vi "AMX-电源尾正面标签1检测参数读取.vi"(7 "error in (no error)":errorcluster caption="错误输入（无错误）", 10 "基路径":path) -> (0 "error out":errorcluster caption="错误输出", 1 "UI电源线尾正面标签1参数":T2={"Rectangle"={"Left"=0, "Top"=0, "Right"=0, "Bottom"=0, "Rotation"=0.0}, "Algorithm "=2, "Parameters"={"Number of Matches Requested"=1, "Minimum Match Score"=800.0, "Angle Ranges"=[{"Start Angle"=-180.0, "End Angle"=180.0}]}, "Advanced Options "=[{"Item"=102, "Value"=10.0}, {"Item"=106, "Value"=300.0}, {"Item"=107, "Value"=0.0}, {"Item"=108, "Value"=6.0}, {"Item"=109, "Value"=1.0}, {"Item"=114, "Value"=25.0}, {"Item"=111, "Value"=20.0}, {"Item"=112, "Value"=10.0}, {"Item"=113, "Value"=20.0}, {"Item"=103, "Value"=1.0}, {"Item"=104, "Value"=20.0}, {"Item"=105, "Value"=0.0}, {"Item"=100, "Value"=5.0}], "模板路径"=path "", "Color Plane "=0} {"Color Plane" items=["Red", "Green", "Blue", "Hue", "Saturation", "Luminance", "Value", "Intensity"]; "Advanced Options"."Item" items=["LD Sampling - Minimum Constrast"=0, "LD Sampling - Enable Subpixel Accuracy"=1, "LD Sampling - Search Strategy"=2, "LD Sampling - Subpixel Iterations"=3, "LD Sampling - Subpixel Tolerance"=4, "LD Sampling - Initial Match List Length"=5, "LD Sampling - Match List Reduction Factor"=6, "LD Sampling - Initial Step Size"=7, "LD Sampling - Intermediate Angular Accuracy"=8, "-"=9, "Pyramid - Max Pyramid Level"=100, "Pyramid - Minimum Contrast"=102, "Pyramid - Enable Subpixel Accuracy"=103, "Pyramid - Subpixel Iterations"=104, "Pyramid - Subpixel Tolerance"=105, "Pyramid - Initial Match List Length"=106, "Pyramid - Match List Reduction Factor"=107, "Pyramid - Intermediate Angular Accuracy"=108, "Pyramid - Process Border Matches"=109, "Pyramid - Min Match Separation Distance"=111, "Pyramid - Min Match Separation Angle"=112, "Pyramid - Max Match Overlap"=113, "Pyramid - Max Cache in MB"=114, "Pyramid - Clear Cache"=115, "-"=116, "Enable Defect Map"=200]; "Algorithm" items=["All", "Low Discrepancy Sampling", "Grayscale Value Pyramid", "Gradients Pyramid"]; "Rectangle"."Rotation" format="%.2f"; "Rectangle"."Left" scale=0.0..1024.0; "Rectangle"."Right" scale=0.0..1024.0}, 2 "UI电源线尾正面标签1基础参数":T3={"IsNorImage"=TRUE, "Exposure Values"=100289, "ImagePath"=path "C:/Users/hedongpo/Desktop/514-hdp/Alignment Assemble System/Test Picture/B/3.bmp"} caption="参数界面" {"Exposure Values" scale=0.0..200000.0})   [LabVIEW 2017]
uses:
  <vilib>/Utility/xml.llb/Read From XML File(string).vi
  Global System.vi
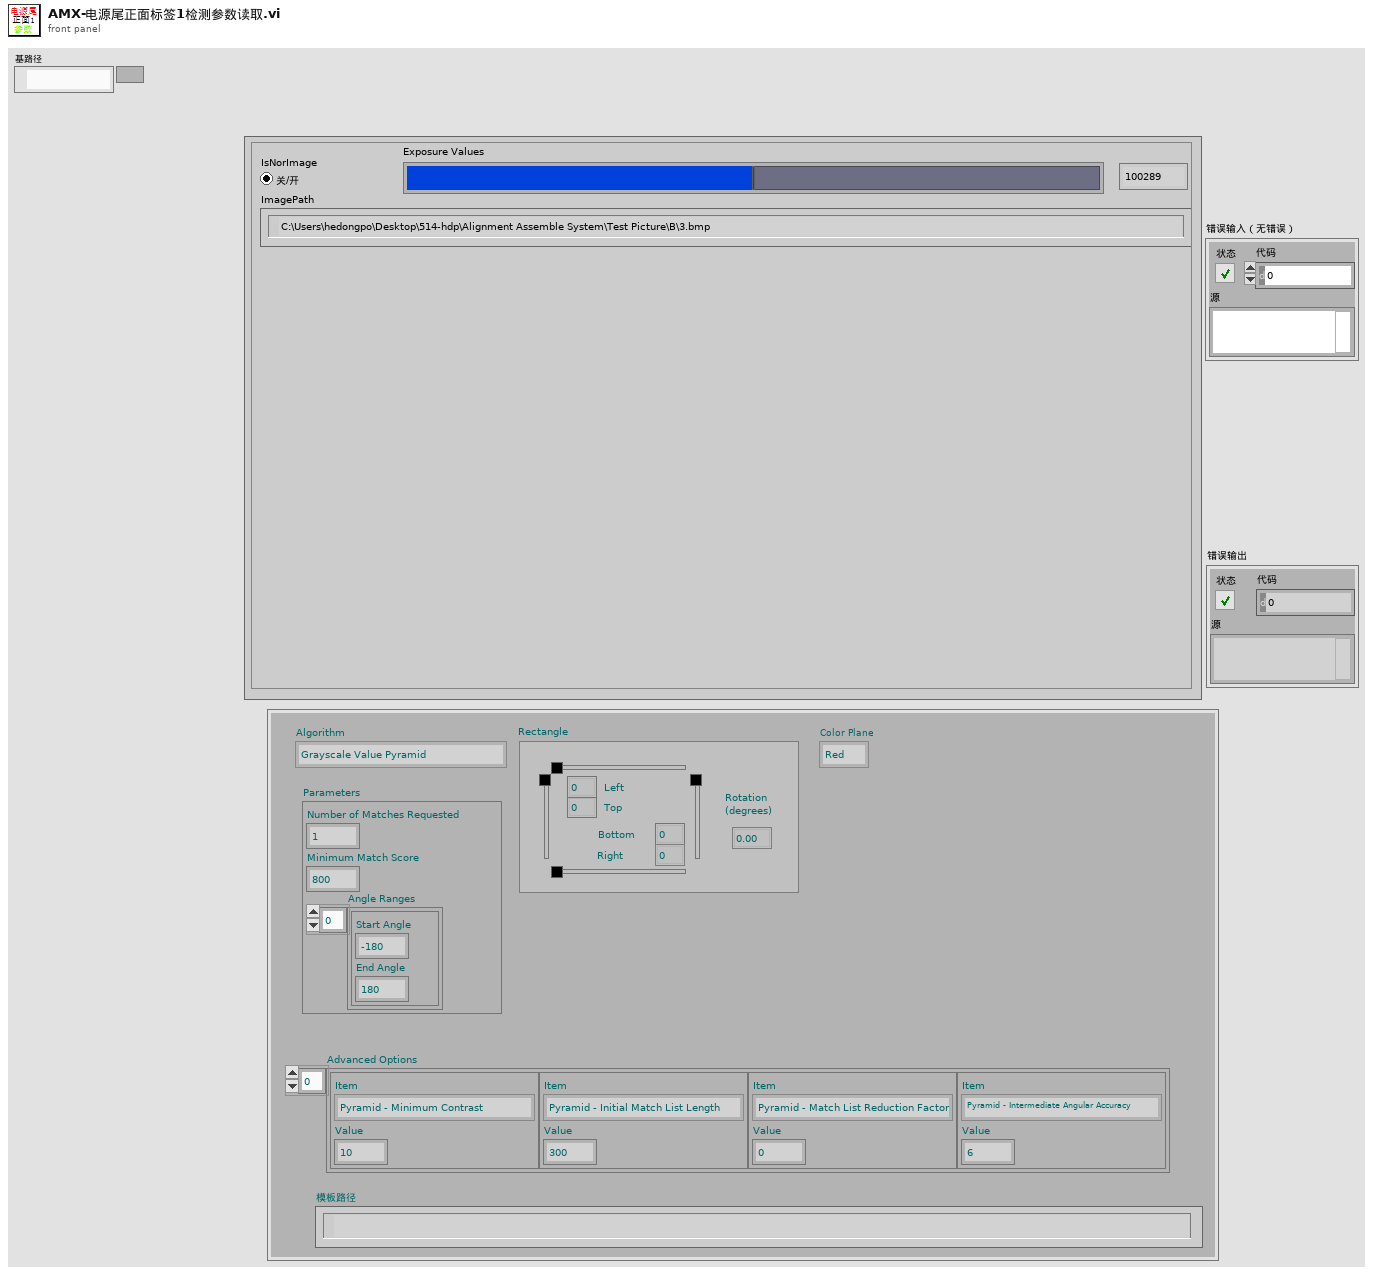
[diagram p1: front panel]
types:
  T1 = typedef "IMAQ Rectangle" = cluster{"Left":i32, "Top":i32, "Right":i32, "Bottom":i32, "Rotation":dbl}
  T2 = cluster{"Rectangle":T1, "Algorithm ":i32, "Parameters":cluster{"Number of Matches Requested":i32, "Minimum Match Score":sgl, "Angle Ranges":cluster{"Start Angle":sgl, "End Angle":sgl}[]}, "Advanced Options ":cluster{"Item":u16, "Value":dbl}[], "模板路径":path, "Color Plane ":i32}
  T3 = cluster{"IsNorImage":bool, "Exposure Values":u32, "ImagePath":path}
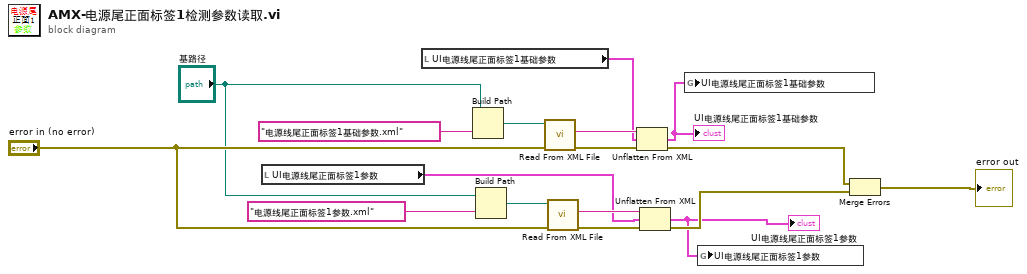
[diagram p0: block diagram]
diagram:
  n1 = local read "UI电源线尾正面标签1参数"() -> (w5:T2)
  n2 = local read "UI电源线尾正面标签1基础参数"() -> (w13:T3)
  n3 = Build Path(base path="基路径", name or relative path="电源线尾正面标签1基础参数.xml" ("名称或相对路径")) -> (appended path=w17:path)
  n4 = Build Path(base path="基路径", name or relative path="电源线尾正面标签1参数.xml" ("名称或相对路径")) -> (appended path=w14:path)
  n5 = call-poly <vilib>:"Read From XML File.vi"("error in (no error)"="error in (no error)", "XML File Path"=w17) -> ("error out"=w11:errorcluster, "XML Elements"=w16:string)  [unwired: 7 in, 1 out]
  n6 = call-poly <vilib>:"Read From XML File.vi"("error in (no error)"="error in (no error)", "XML File Path"=w14) -> ("error out"=w9:errorcluster, "XML Elements"=w15:string)  [unwired: 7 in, 1 out]
  n7 = Unflatten From XML(xml string=w16, type=w13, error in (no error)=w11) -> (value=w2:T3, error out=w10:errorcluster)
  "UI电源线尾正面标签1基础参数" <- w2
  n8 = Unflatten From XML(xml string=w15, type=w5, error in (no error)=w9) -> (value=w1:T2, error out=w8:errorcluster)
  "UI电源线尾正面标签1参数" <- w1
  n9 = global write "Global System.vi" "UI电源线尾正面标签1基础参数"(w2) -> ()
  n10 = global write "Global System.vi" "UI电源线尾正面标签1参数"(w1) -> ()
  n11 = Merge Errors(w10, w8) -> (→"error out":errorcluster)
